vi "AddParser.vi"(8 "error in (no error)":errorcluster, 10 "ParserConfig":refnum<class "ParserConfig.lvclass">, 11 "ArgumentParser in":refnum<class "ArgumentParser.lvclass">) -> (0 "error out":errorcluster, 3 "ArgumentParser out":refnum<class "ArgumentParser.lvclass">)   [LabVIEW 2022 SP3, in "ArgumentParser.lvlib" / "ArgumentParser.lvclass"]
uses:
  ArgumentParser.lvclass
  ParserConfig/ParserConfig.lvclass
  ParserConfig/ParserConfig.lvclass/ParserConfig.ctl
  ArgumentParser.lvclass/ArgumentParser.ctl
  ParserConfig/Read Name.vi
  ParserConfig/Read Aliases.vi
  ParserConfig/Read Usage.vi
  ParserConfig/Read Description.vi
  ParserConfig/Read Epilog.vi
  ParserConfig/Read PrefixCharacters.vi
  ParserConfig/Read FromFilePrefixCharacters.vi
  ParserConfig/Read ArgumentDefault.vi
  ParserConfig/Read ConflictHandler.vi
  ParserConfig/Read AddHelp.vi
  ParserConfig/Read AllowAbbreviation.vi
  ParserConfig/Read ExitOnError.vi
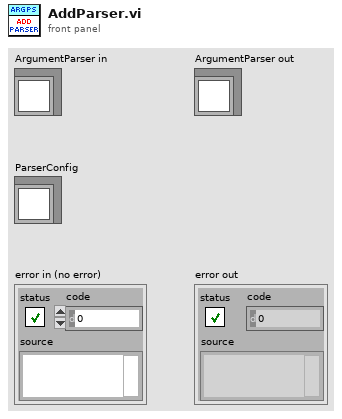
[diagram p1: front panel]
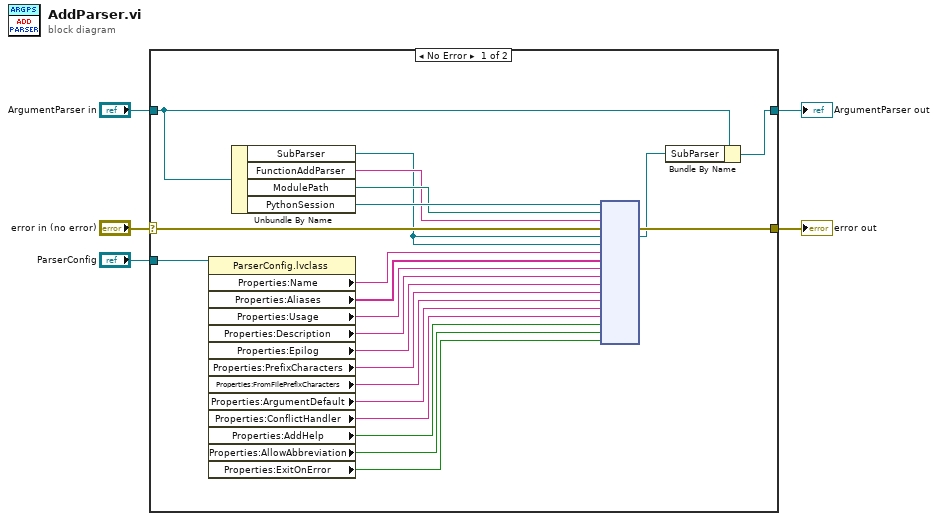
[diagram p0: block diagram]
diagram:
  n1 = case shown="No Error" "error in (no error)" {
    selector: "error in (no error)" -> [w27 w29]
    tunnel: [w26 w29] -> w2
    tunnel: [w11 w28] -> w4
    tunnel: "ArgumentParser in" -> [w10 w28]
    tunnel: "ParserConfig" -> [w9 _]
    frame No Error {
      n2 = property class="ParserConfig.lvclass"(reference=w9) -> ("Properties:Name"=w22:string, "Properties:Aliases"=w21:string[], "Properties:Usage"=w20:string, "Properties:Description"=w19:string, "Properties:Epilog"=w18:string, "Properties:PrefixCharacters"=w17:string, "Properties:FromFilePrefixCharacters"=w8:string, "Properties:ArgumentDefault"=w16:string, "Properties:ConflictHandler"=w15:string, "Properties:AddHelp"=w14:bool, "Properties:AllowAbbreviation"=w6:bool, "Properties:ExitOnError"=w7:bool)  [unwired: 1 in, 2 out]
      n3 = Unbundle By Name(w10) -> ("SubParser"=w13:refnum<k38>, "FunctionAddParser"=w23:string, "ModulePath"=w24:path, "PythonSession"=w25:refnum<k35>)
      n4 = node(w25, w24, w23, w27, w13, w13, w22, w21, w20, w19, w18, w17, w8, w16, w15, w14, w6, w7) -> (w26:errorcluster, w12:refnum<k38>)  [unwired: 13 in, 3 out]
      n5 = Bundle By Name(cluster=w10, "SubParser"=w12) -> (w11:refnum<class "ArgumentParser.lvclass">)
    }
    frame Error {
    }
  }
  "error out" <- w2
  "ArgumentParser out" <- w4
